vi "Test HighFrequency Client Connection.vi"() -> ()   [LabVIEW 2013]
uses:
  Control Packets/CONNACK/Connect Return Code -- enum.ctl
  Server class/Server.lvclass/Server.ctl
  Client/Client.lvclass/Client.ctl
  Control Packets/PUBLISH/PUBLISH.lvclass
  Server class/Server.lvclass
  MQTT_Base/MQTT_Base.lvclass
  Client/Client.lvclass
  Control Packets/CONNACK/CONNACK.lvclass
panel:
  out "NO RESPONSE":bool
  out "timed out?":bool
  out "Stop":dbl format="%.06f"
  out "Connect":dbl format="%.06f"
  out "Start":dbl format="%.06f"
  out "STOPPING":bool
  out "Waveform Chart":T1(graph)
  out "Loop period (s)":dbl format="%.06f"
  out "client Outgoing ID Request":i32
  out "Process Response":i32
  out "Process Incoming ID Request":i32
  out "Process Status":T2=enum."Server Unavailable"
  out "error server":errorcluster
  out "Client Status":T2=enum."Server Unavailable"
  out "error client process":errorcluster
  out "NbConnections":u32
  out "error client consumer":errorcluster
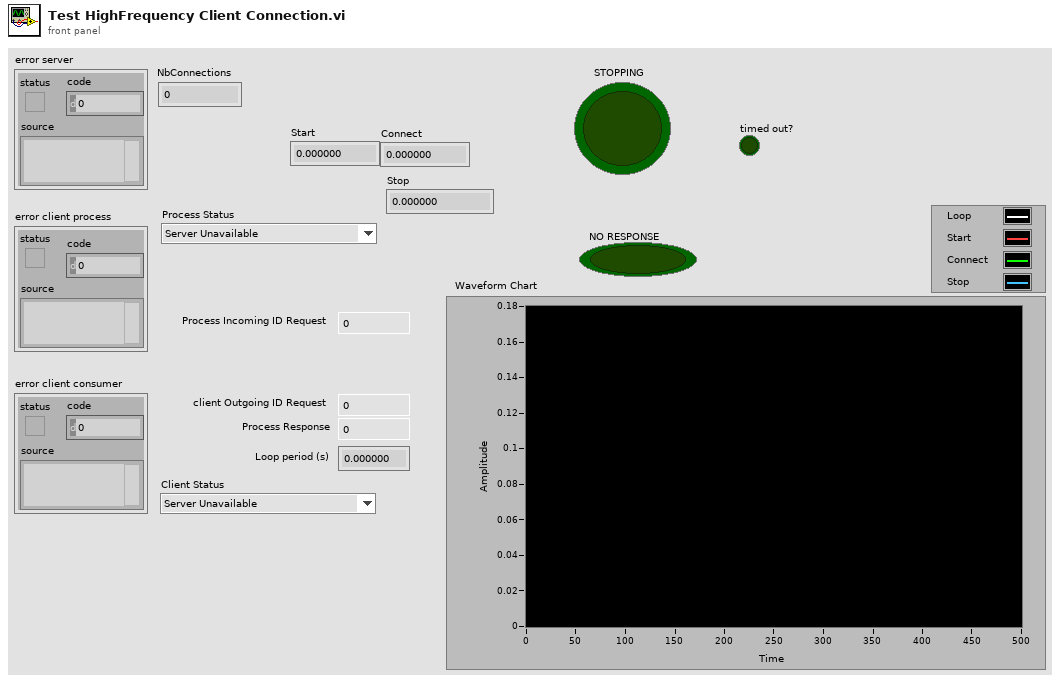
[diagram p1: front panel]
types:
  T1 = cluster{dbl, "elapsed (s)":dbl, "elapsed (s)":dbl, "elapsed (s)":dbl}
  T2 = typedef "CONNACK.lvclass/Connect Return Code -- enum.ctl" = enum16{"Connection accepted", "Unacceptable protocol version", "Identifier Rejected", "Server Unavailable", "Bad Username or Password", "Not Authorized"}
  T3 = typedef "MQTT Server.lvlib/Server.lvclass/Public Events -- cluster.ctl" = cluster{"NbConnections":refnum<user-event>}
  T4 = typedef "MQTT Server.lvlib/Client.lvclass/Public Events -- cluster.ctl" = cluster{"Connection Status":refnum<user-event>, "Connected":refnum<user-event>, "Application Message":refnum<user-event>}
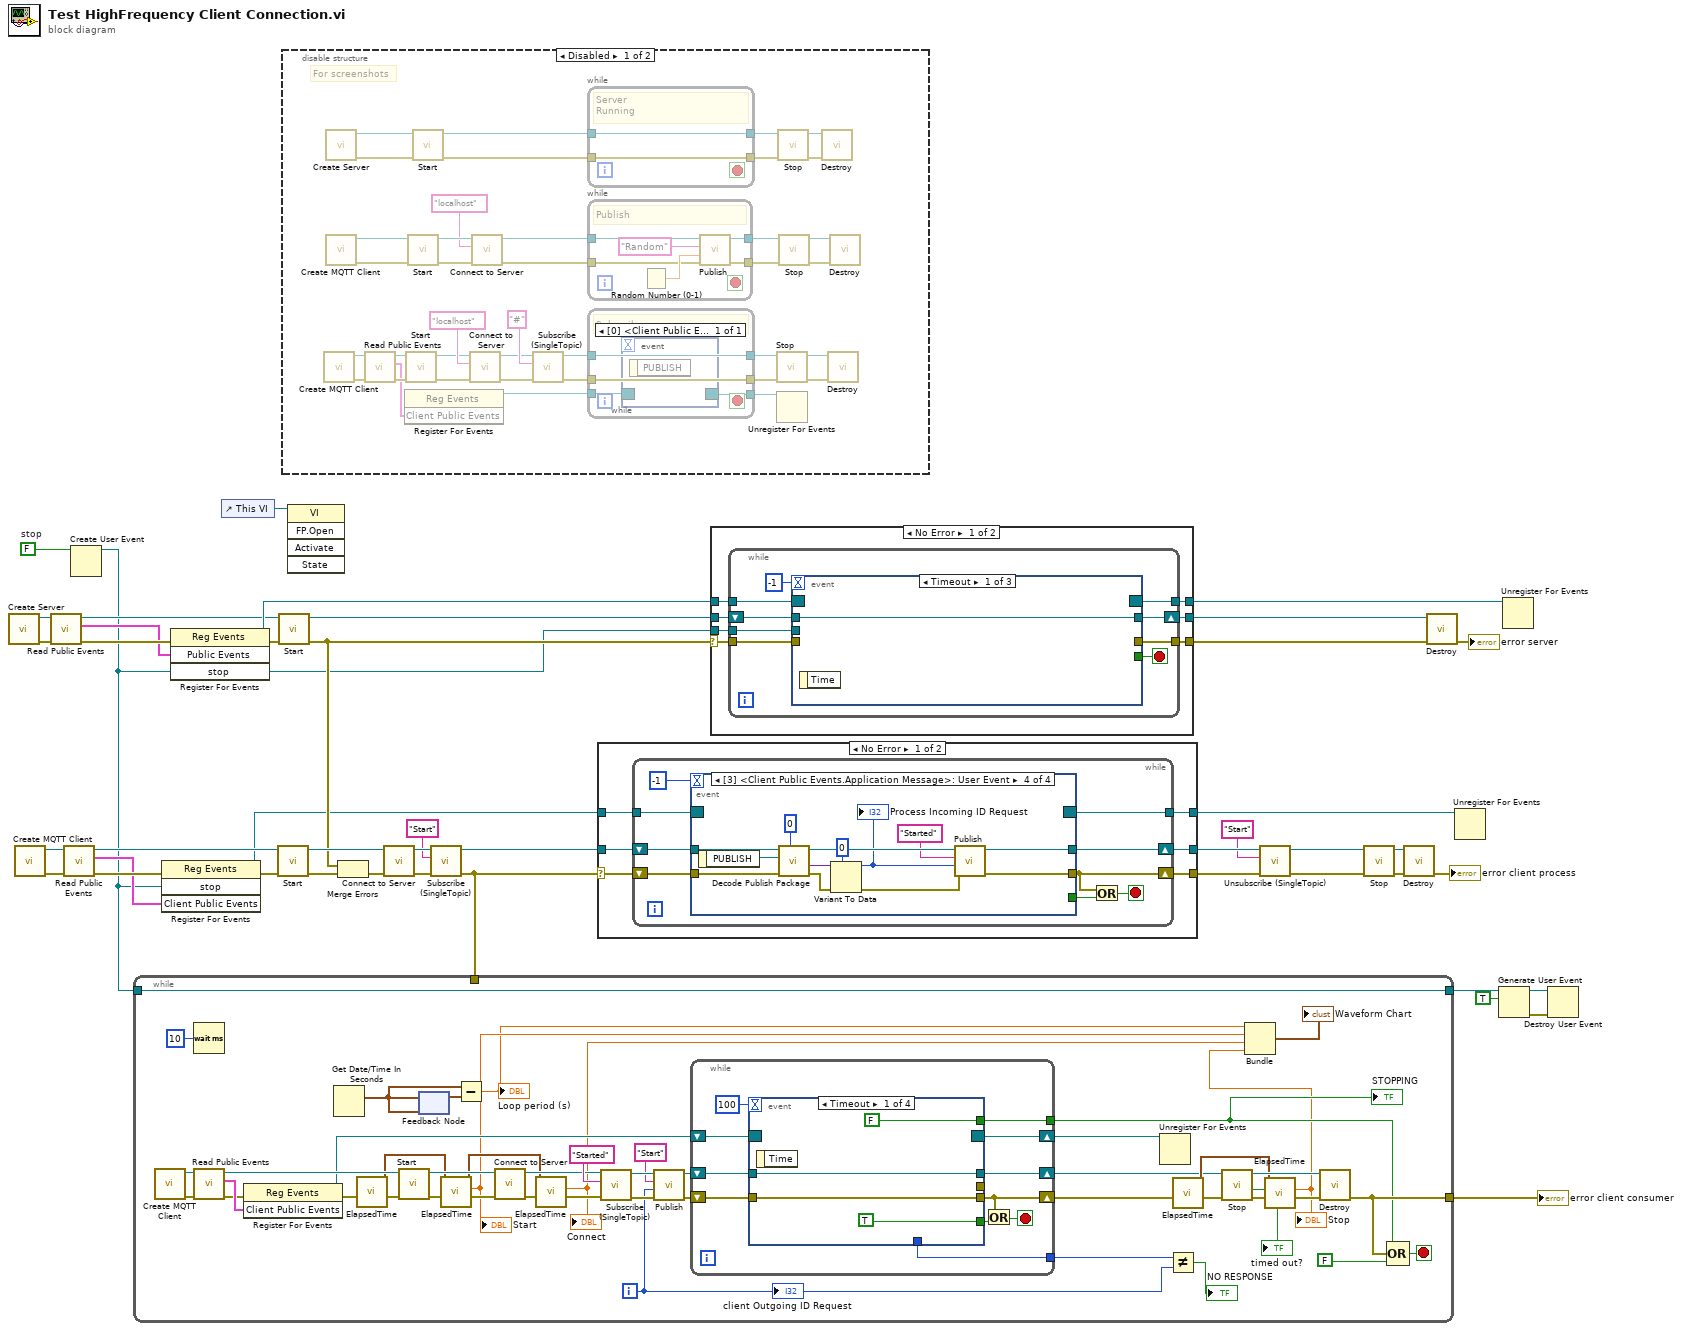
[diagram p0: block diagram]
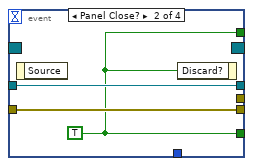
[diagram p2: hidden frame]
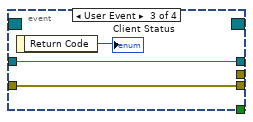
[diagram p3: hidden frame]
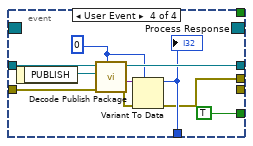
[diagram p4: hidden frame]
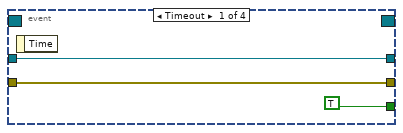
[diagram p5: hidden frame]
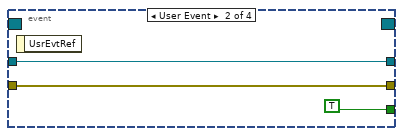
[diagram p6: hidden frame]
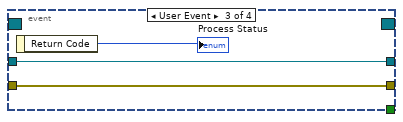
[diagram p7: hidden frame]
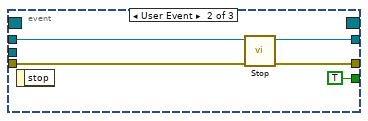
[diagram p10: hidden frame]
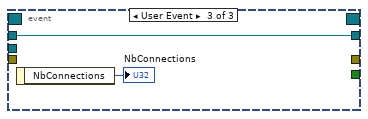
[diagram p11: hidden frame]
diagram:
  w28 = FALSE  # stop
  n1 = call "Create Server.vi"() -> ("error out"=w43:errorcluster, "Server"=w44:refnum<class "Server.lvclass">)  [unwired: 10 in]
  n2 = call "Create MQTT Client.vi"() -> ("error out"=w33:errorcluster, "Client out"=w32:refnum<class "Client.lvclass">)  [unwired: 10 in]
  n3 = call "Read Public Events.vi"("error in (no error)"=w43, "Server in"=w44) -> ("error out"=w42:errorcluster, "Public Events"=w41:T3, "Server out"=w38:refnum<class "Server.lvclass">)  [unwired: 7 in]
  n4 = call "Read Public Events.vi"("error in (no error)"=w33, "Client in"=w32) -> ("error out"=w27:errorcluster, "Client Public Events"=w25:T4, "Client out"=w31:refnum<class "Client.lvclass">)  [unwired: 7 in]
  n5 = Create User Event(user event datatype=w28) -> (user event=w5:refnum<user-event>)  [unwired: 1 in, 1 out]
  n6 = register-events(error in=w27, w5, w25) -> (reference out=w17:refnum<event-registration>, error out=w26:errorcluster)  [unwired: 1 in]
  n7 = register-events(error in=w42, w41, w5) -> (reference out=w40:refnum<event-registration>, error out=w36:errorcluster)  [unwired: 1 in]
  n8 = control-ref of="This VI"() -> (w24:refnum<vi>)
  n9 = call "Start.vi"("error in (no error)"=w26, "MQTT_Base in"=w31) -> ("error out"=w29:errorcluster, "MQTT_Base out"=w30:refnum<class "Client.lvclass">)  [unwired: 7 in, 1 out]
  n10 = call "Start.vi"("error in (no error)"=w36, "MQTT_Base in"=w38) -> ("error out"=w22:errorcluster, "MQTT_Base out"=w37:refnum<class "Server.lvclass">)  [unwired: 7 in, 1 out]
  n11 = disable-structure shown="Disabled" {
    frame Disabled {
      # "For screenshots"
      n12 = call "Create MQTT Client.vi"() -> ("error out"=w50:errorcluster, "Client out"=w52:refnum<class "Client.lvclass">)  [unwired: 10 in]
      n13 = call "Create Server.vi"() -> ("error out"=w77:errorcluster, "Server"=w76:refnum<class "Server.lvclass">)  [unwired: 10 in]
      n14 = call "Create MQTT Client.vi"() -> ("error out"=w74:errorcluster, "Client out"=w75:refnum<class "Client.lvclass">)  [unwired: 10 in]
      n15 = call "Read Public Events.vi"("error in (no error)"=w50, "Client in"=w52) -> ("error out"=w49:errorcluster, "Client Public Events"=w48:T4, "Client out"=w51:refnum<class "Client.lvclass">)  [unwired: 7 in]
      n16 = register-events(w48) -> (reference out=w47:refnum<event-registration>)  [unwired: 2 in, 1 out]
      n17 = call "Start.vi"("error in (no error)"=w49, "MQTT_Base in"=w51) -> ("error out"=w67:errorcluster, "MQTT_Base out"=w68:refnum<class "Client.lvclass">)  [unwired: 7 in, 1 out]
      n18 = call "Start.vi"("error in (no error)"=w74, "MQTT_Base in"=w75) -> ("error out"=w81:errorcluster, "MQTT_Base out"=w80:refnum<class "Client.lvclass">)  [unwired: 7 in, 1 out]
      n19 = call "Start.vi"("error in (no error)"=w77, "MQTT_Base in"=w76) -> ("error out"=w59:errorcluster, "MQTT_Base out"=w61:refnum<class "Server.lvclass">)  [unwired: 7 in, 1 out]
      n20 = call "Connect to Server.vi"("error in (no error)"=w67, "address (localhost)"="localhost" ("Topic Filter"), "Client in"=w68) -> ("error out"=w55:errorcluster, "Client out"=w56:refnum<class "Client.lvclass">)  [unwired: 5 in, 2 out]
      n21 = call "Connect to Server.vi"("error in (no error)"=w81, "address (localhost)"="localhost" ("Topic Filter"), "Client in"=w80) -> ("error out"=w63:errorcluster, "Client out"=w66:refnum<class "Client.lvclass">)  [unwired: 5 in, 2 out]
      n22 = call "Subscribe (SingleTopic).vi"("error in (no error)"=w55, "Topic Filter"="#", "MQTT_Base in"=w56) -> ("error out"=w53:errorcluster, "MQTT_Base out"=w54:refnum<class "Client.lvclass">)  [unwired: 7 in]
      n23 = while {
        tunnel: [w95] -> w62
        tunnel: w61 -> [w95]
        tunnel: w59 -> [w94]
        tunnel: [w94] -> w60
        stop <- _ stop-if-true
        # "Server\nRunning"
      }
      n24 = while {
        tunnel: w66 -> [w91]
        tunnel: [w90] -> w65
        tunnel: [w89] -> w64
        tunnel: w63 -> [w88]
        stop <- _ stop-if-true
        # "Publish"
        n25 = Random Number (0-1)() -> (number: 0 to 1=w93:dbl)
        n26 = call "Publish.vi"("error in (no error)"=w88, "Payload"=w93, "Topic Name (empty: Payload name)"="Random", "Client in"=w91) -> ("error out"=w89:errorcluster, "Client out"=w90:refnum<class "Client.lvclass">)  [unwired: 5 in, 1 out]
      }
      n27 = while {
        tunnel: [w87] -> w57
        tunnel: w54 -> [w87]
        tunnel: w53 -> [w86]
        tunnel: [w86] -> w58
        tunnel: w47 -> [w85]
        tunnel: [w84] -> w46
        stop <- _ stop-if-true
        # "Subscribe"
        n28 = event shown="[0] <Client Public Events.Application Message>: User Event" {
          selector: w85 -> [_]
          dyn-events: [_] -> w84
          timeout: _ -> [_]
          event User Event {
            n29 = event-data() -> ()  [unwired: 1 in, 1 out]
          }
        }
      }
      n30 = call "Stop.vi"("error in (no error)"=w58, "MQTT_Base in"=w57) -> ("error out"=w70:errorcluster, "MQTT_Base out"=w71:refnum<class "Client.lvclass">)  [unwired: 7 in, 1 out]
      n31 = Unregister For Events(event registration refnum=w46) -> ()  [unwired: 1 in, 1 out]
      n32 = call "Stop.vi"("error in (no error)"=w60, "MQTT_Base in"=w62) -> ("error out"=w83:errorcluster, "MQTT_Base out"=w82:refnum<class "Server.lvclass">)  [unwired: 7 in, 1 out]
      n33 = call "Stop.vi"("error in (no error)"=w64, "MQTT_Base in"=w65) -> ("error out"=w79:errorcluster, "MQTT_Base out"=w78:refnum<class "Client.lvclass">)  [unwired: 7 in, 1 out]
      n34 = call "Destroy.vi"("error in (no error)"=w83, "MQTT_Base in"=w82) -> ()  [unwired: 8 in, 2 out]
      n35 = call "Destroy.vi"("error in (no error)"=w70, "MQTT_Base in"=w71) -> ()  [unwired: 8 in, 2 out]
      n36 = call "Destroy.vi"("error in (no error)"=w79, "MQTT_Base in"=w78) -> ()  [unwired: 8 in, 2 out]
    }
    frame Enabled {
    }
  }
  n37 = invoke class="VI" method="FP.Open"(reference=w24) -> ()  [unwired: 4 in, 5 out]
  n38 = Merge Errors(w22, w29) -> (w34:errorcluster)
  n39 = call "Connect to Server.vi"("error in (no error)"=w34, "Client in"=w30) -> ("error out"=w20:errorcluster, "Client out"=w21:refnum<class "Client.lvclass">)  [unwired: 6 in, 2 out]
  n40 = call "Subscribe (SingleTopic).vi"("error in (no error)"=w20, "Topic Filter"="Start", "MQTT_Base in"=w21) -> ("error out"=w6:errorcluster, "MQTT_Base out"=w18:refnum<class "Client.lvclass">)  [unwired: 7 in]
  n41 = while {
    tunnel: [w124] -> w7
    tunnel: w6 -> [_]
    tunnel: [w122] -> w4
    tunnel: w5 -> [w122]
    i -> [w123]
    stop <- w125 stop-if-true
    n42 = call "Create MQTT Client.vi"() -> ("error out"=w141:errorcluster, "Client out"=w142:refnum<class "Client.lvclass">)  [unwired: 10 in]
    n43 = Wait (ms)(milliseconds to wait=u32 10) -> ()  [unwired: 1 out]
    n44 = call "Read Public Events.vi"("error in (no error)"=w141, "Client in"=w142) -> ("error out"=w136:errorcluster, "Client Public Events"=w137:T4, "Client out"=w140:refnum<class "Client.lvclass">)  [unwired: 7 in]
    n45 = register-events(error in=w136, w137) -> (reference out=w135:refnum<event-registration>, error out=w118:errorcluster)  [unwired: 1 in]
    n46 = Get Date/Time In Seconds() -> (seconds since 1Jan1904=w120:timestamp)
    n47 = call "ElapsedTime.vi"("error in"=w118) -> ("error out"=w117:errorcluster, "current time"=w114:timestamp)  [unwired: 8 in, 1 out]
    n48 = call "Start.vi"("error in (no error)"=w117, "MQTT_Base in"=w140) -> ("error out"=w115:errorcluster, "MQTT_Base out"=w139:refnum<class "Client.lvclass">)  [unwired: 7 in, 1 out]
    n49 = feedback-in #1(w120) -> ()
    n50 = feedback #1(w120) -> (w121:timestamp)
    n51 = call "ElapsedTime.vi"("error in"=w115, "compare time"=w114) -> ("error out"=w116:errorcluster, "elapsed (s)"=w106:dbl, "current time"=w111:timestamp)  [unwired: 7 in]
    "Start" <- w106
    n52 = Subtract(x=w120, y=w121) -> (x-y=w103:dbl)
    "Loop period (s)" <- w103
    n53 = call "Connect to Server.vi"("error in (no error)"=w116, "Client in"=w139) -> ("error out"=w113:errorcluster, "Client out"=w132:refnum<class "Client.lvclass">)  [unwired: 6 in, 2 out]
    n54 = call "ElapsedTime.vi"("error in"=w113, "compare time"=w111) -> ("error out"=w112:errorcluster, "elapsed (s)"=w105:dbl)  [unwired: 7 in, 1 out]
    "Connect" <- w105
    n55 = call "Subscribe (SingleTopic).vi"("error in (no error)"=w112, "Topic Filter"="Started", "MQTT_Base in"=w132) -> ("error out"=w131:errorcluster, "MQTT_Base out"=w130:refnum<class "Client.lvclass">)  [unwired: 7 in]
    n56 = call "Publish.vi"("error in (no error)"=w131, "Payload"=w123, "Topic Name (empty: Payload name)"="Start" ("Topic Filter"), "Client in"=w130) -> ("error out"=w128:errorcluster, "Client out"=w129:refnum<class "Client.lvclass">)  [unwired: 5 in, 1 out]
    n57 = while {
      shift-right: [w151] -> w100
      shift-left: w129 -> [w147]
      shift-right: [w152] -> w134
      shift-left: w135 -> [w153]
      shift-right: [w150] -> w99
      shift-left: w128 -> [w146]
      tunnel: [w144] -> w126
      tunnel: [w143] -> w119
      stop <- w145 stop-if-true
      n58 = event shown="[0] Timeout" {
        selector: w153 -> [_ _ _ _]
        dyn-events: [_ _ _ _] -> w152
        timeout: 100 -> [_ _ _ _]
        tunnel: w147 -> [w156 w160 w162 w172]
        tunnel: [w156 w160 w162 w170] -> w151
        tunnel: [w155 w159 w161 _] -> w150
        tunnel: w146 -> [w155 w159 w161 w169]
        tunnel: [TRUE w158 _ TRUE] -> w149
        tunnel: [_ _ _ w165] -> w144
        tunnel: [FALSE w158 _ _] -> w143
        tunnel: [_ _ _ w164] -> _
        event Timeout {
          n59 = event-data() -> ()  [unwired: 1 in, 1 out]
        }
        event Panel Close? {
          w158 = TRUE
          n60 = event-data() -> ()  [unwired: 1 in, 1 out]
          n61 = event-data("Discard?"=w158) -> ()  [unwired: 1 in, 1 out]
        }
        event User Event {
          n62 = event-data() -> ("Return Code"=→"Client Status":T2)  [unwired: 1 in]
        }
        event User Event {
          w168 = 0
          n63 = event-data() -> ("PUBLISH"=w173:refnum<class "PUBLISH.lvclass">)  [unwired: 1 in]
          n64 = call "Decode Publish Package.vi"("Type"=w168, "error in (no error)"=w169, "PUBLISH in"=w173, "MQTT_Base in"=w172) -> ("error out"=w167:errorcluster, "Payload"=w171:variant, "MQTT_Base out"=w170:refnum<class "Client.lvclass">)  [unwired: 4 in, 1 out]
          n65 = Variant To Data(error in=w167, type=w168, Variant=w171) -> (data=w165:i32, error out=w164:errorcluster)
          "Process Response" <- w165
        }
      }
      n66 = Or(x=w150, y=w149) -> (x .or. y?=w145:bool)
    }
    "STOPPING" <- w119
    n67 = Unregister For Events(event registration refnum=w134) -> ()  [unwired: 1 in, 1 out]
    n68 = Not Equal?(x=w126, y=w123) -> (x != y?=→"NO RESPONSE":bool)
    n69 = call "ElapsedTime.vi"("error in"=w99) -> ("error out"=w110:errorcluster, "current time"=w107:timestamp)  [unwired: 8 in, 1 out]
    n70 = call "Stop.vi"("error in (no error)"=w110, "MQTT_Base in"=w100) -> ("error out"=w108:errorcluster, "timed out?"=→"timed out?":bool, "MQTT_Base out"=w138:refnum<class "Client.lvclass">)  [unwired: 7 in]
    n71 = call "ElapsedTime.vi"("error in"=w108, "compare time"=w107) -> ("error out"=w109:errorcluster, "elapsed (s)"=w104:dbl)  [unwired: 7 in, 1 out]
    "Stop" <- w104
    n72 = Bundle(w103, "elapsed (s)"=w106, "elapsed (s)"=w105, "elapsed (s)"=w104) -> (→"Waveform Chart":T1)  [unwired: 1 in]
    n73 = call "Destroy.vi"("error in (no error)"=w109, "MQTT_Base in"=w138) -> ("error out"=w124:errorcluster)  [unwired: 8 in, 1 out]
    n74 = Compound Arithmetic op=OR(w119, w124, FALSE) -> (w125:bool)
    "client Outgoing ID Request" <- w123
  }
  "error client consumer" <- w7
  n75 = case shown="No Error" w6 {
    selector: w6 -> [w174 w211]
    tunnel: w17 -> [w179 w213]
    tunnel: [w178 w213] -> w13
    tunnel: w18 -> [w177 w212]
    tunnel: [w176 w212] -> w11
    tunnel: [w175 w211] -> w9
    frame No Error {
      n76 = while {
        tunnel: w179 -> [w188]
        tunnel: [w187] -> w178
        shift-right: [w185] -> w176
        shift-left: w177 -> [w186]
        shift-right: [w182] -> w175
        shift-left: w174 -> [w184]
        stop <- w183 stop-if-true
        n77 = event shown="[3] <Client Public Events.Application Message>: User Event" {
          selector: w188 -> [_ _ _ _]
          dyn-events: [_ _ _ _] -> w187
          timeout: -1 -> [_ _ _ _]
          tunnel: w186 -> [w190 w193 w196 w209]
          tunnel: [w190 w193 w196 w202] -> w185
          tunnel: [w189 w192 w195 w198] -> w182
          tunnel: w184 -> [w189 w192 w195 w206]
          tunnel: [TRUE TRUE _ _] -> w181
          event Timeout {
            n78 = event-data() -> ()  [unwired: 1 in, 1 out]
          }
          event User Event {
            n79 = event-data() -> ()  [unwired: 1 in, 1 out]
          }
          event User Event {
            n80 = event-data() -> ("Return Code"=→"Process Status":T2)  [unwired: 1 in]
          }
          event User Event {
            n81 = event-data() -> ("PUBLISH"=w210:refnum<class "PUBLISH.lvclass">)  [unwired: 1 in]
            n82 = call "Decode Publish Package.vi"("Type"=0, "error in (no error)"=w206, "PUBLISH in"=w210, "MQTT_Base in"=w209) -> ("error out"=w205:errorcluster, "Payload"=w208:variant, "MQTT_Base out"=w203:refnum<class "Client.lvclass">)  [unwired: 4 in, 1 out]
            n83 = Variant To Data(error in=w205, type=0, Variant=w208) -> (data=w200:i32, error out=w199:errorcluster)
            "Process Incoming ID Request" <- w200
            n84 = call "Publish.vi"("error in (no error)"=w199, "Payload"=w200, "Topic Name (empty: Payload name)"="Started" ("Topic Filter"), "Client in"=w203) -> ("error out"=w198:errorcluster, "Client out"=w202:refnum<class "Client.lvclass">)  [unwired: 5 in, 1 out]
          }
        }
        n85 = Or(x=w182, y=w181) -> (x .or. y?=w183:bool)
      }
    }
    frame Error {
    }
  }
  n86 = case shown="No Error" w22 {
    selector: w22 -> [w214 w238]
    tunnel: w37 -> [w220 w240]
    tunnel: [w219 w240] -> w45
    tunnel: w40 -> [w218 w239]
    tunnel: [w217 w239] -> w39
    tunnel: [w216 w238] -> w35
    tunnel: w5 -> [w215 _]
    frame No Error {
      n87 = while {
        shift-right: [w226] -> w219
        shift-left: w220 -> [w228]
        tunnel: w218 -> [w225]
        tunnel: [w224] -> w217
        tunnel: [w223] -> w216
        tunnel: w215 -> [w222]
        tunnel: w214 -> [w221]
        stop <- w227 stop-if-true
        n88 = event shown="[0] Timeout" {
          selector: w225 -> [_ _ _]
          dyn-events: [_ _ _] -> w224
          timeout: -1 -> [_ _ _]
          tunnel: w228 -> [w230 w235 w237]
          tunnel: [_ TRUE ("Discard?") _] -> w227
          tunnel: [w230 w234 w237] -> w226
          tunnel: [_ w233 _] -> w223
          tunnel: w222 -> [_ _ _]
          tunnel: w221 -> [_ w231 _]
          event Timeout {
            n89 = event-data() -> ()  [unwired: 1 in, 1 out]
          }
          event User Event {
            n90 = event-data() -> ()  [unwired: 1 in, 1 out]
            n91 = call "Stop.vi"("error in (no error)"=w231, "MQTT_Base in"=w235) -> ("error out"=w233:errorcluster, "MQTT_Base out"=w234:refnum<class "Server.lvclass">)  [unwired: 7 in, 1 out]
          }
          event User Event {
            n92 = event-data() -> ("NbConnections"=→"NbConnections":u32)  [unwired: 1 in]
          }
        }
      }
    }
    frame Error {
    }
  }
  n93 = call "Unsubscribe (SingleTopic).vi"("error in (no error)"=w9, "Topic Filter"="Start", "MQTT_Base in"=w11) -> ("error out"=w10:errorcluster, "MQTT_Base out"=w12:refnum<class "Client.lvclass">)  [unwired: 7 in]
  n94 = call "Stop.vi"("error in (no error)"=w10, "MQTT_Base in"=w12) -> ("error out"=w15:errorcluster, "MQTT_Base out"=w16:refnum<class "Client.lvclass">)  [unwired: 7 in, 1 out]
  n95 = call "Destroy.vi"("error in (no error)"=w15, "MQTT_Base in"=w16) -> ("error out"=→"error client process":errorcluster)  [unwired: 8 in, 1 out]
  n96 = call "Destroy.vi"("error in (no error)"=w35, "MQTT_Base in"=w45) -> ("error out"=→"error server":errorcluster)  [unwired: 8 in, 1 out]
  n97 = Unregister For Events(event registration refnum=w13) -> ()  [unwired: 1 in, 1 out]
  n98 = Generate User Event(user event=w4, event data cluster=TRUE ("event data")) -> (user event out=w2:refnum<user-event>, error out=w3:errorcluster)  [unwired: 2 in]
  n99 = Unregister For Events(event registration refnum=w39) -> ()  [unwired: 1 in, 1 out]
  n100 = Destroy User Event(user event=w2, error in=w3) -> ()  [unwired: 1 out]
